vi "02-调小程序.vi"() -> ()   [LabVIEW 2015]
panel:
  out "数组":i32[](array[numeric])
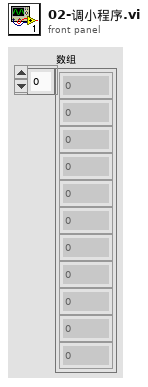
[diagram p1: front panel]
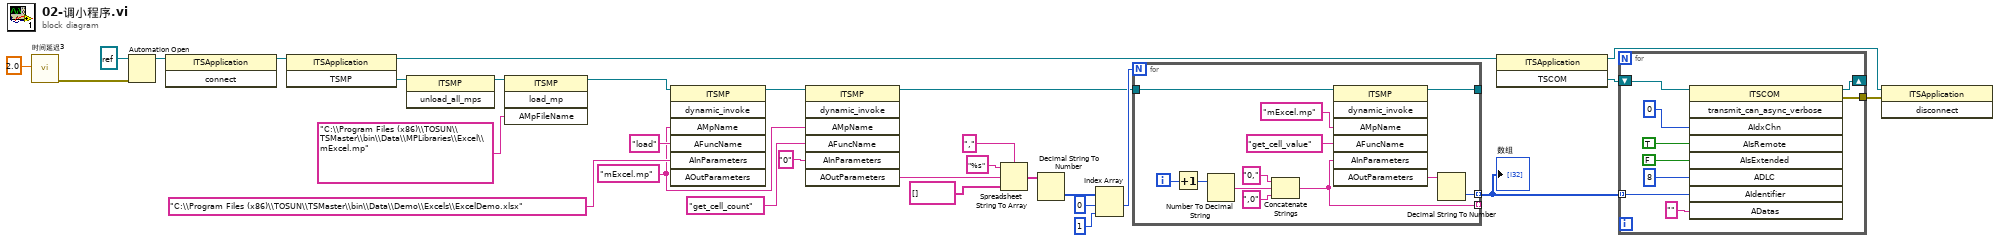
[diagram p0: block diagram]
diagram:
  w3 = "mExcel.mp" ("AMpName")
  n1 = call "时间延迟3"("Delay Time (s)"=2.0) -> ("error out"=w28:errorcluster)  [unwired: 10 in]
  n2 = Automation Open(error in (no error)=w28, Automation Refnum=refnum<k7> refnum ("TSMaster.ITSApplication")) -> (Automation Refnum=w27:refnum<k7>)  [unwired: 2 in, 1 out]
  n3 = invoke on="调用节点" class="ITSApplication" method="connect"(reference=w27) -> (reference out=w4:refnum<k7>)  [unwired: 2 in, 2 out]
  n4 = invoke on="调用节点" class="ITSApplication" method="TSMP"(reference=w4) -> (reference out=w6:refnum<k7>, "TSMP"=w23:refnum<k7>)  [unwired: 2 in, 1 out]
  n5 = invoke on="调用节点" class="ITSMP" method="unload_all_mps"(reference=w23) -> (reference out=w22:refnum<k7>)  [unwired: 2 in, 2 out]
  n6 = invoke on="调用节点" class="ITSMP" method="load_mp"(reference=w22, "AMpFileName"="C:\\Program Files (x86)\\TOSUN\\TSMaster\\bin\\Data\\MPLibraries\\Excel\\mExcel.mp") -> (reference out=w1:refnum<k7>)  [unwired: 2 in, 3 out]
  n7 = invoke on="调用节点" class="ITSMP" method="dynamic_invoke"(reference=w1, "AMpName"=w3, "AFuncName"="load", "AInParameters"="C:\\Program Files (x86)\\TOSUN\\TSMaster\\bin\\Data\\Demo\\Excels\\ExcelDemo.xlsx") -> (reference out=w2:refnum<k7>)  [unwired: 3 in, 6 out]
  n8 = invoke on="调用节点" class="ITSMP" method="dynamic_invoke"(reference=w2, "AMpName"=w3, "AFuncName"="get_cell_count", "AInParameters"="0") -> (reference out=w8:refnum<k7>, "AOutParameters"=w17:string)  [unwired: 3 in, 5 out]
  n9 = Spreadsheet String To Array(delimiter (Tab)="," ("分隔符(Tab)"), format string="%s" ("格式字符串"), spreadsheet string=w17, array type (2D Dbl)=string[] []) -> (array=w13:string[])
  n10 = Decimal String To Number(string=w13) -> (number=w12:i32[])  [unwired: 2 in, 1 out]
  n11 = Index Array(array=w12, index #1=0 ("索引"), index #2=1 ("索引")) -> (element #1=w9:i32)  [unwired: 1 out]
  n12 = for {
    N: w9 -> [_]
    tunnel: w8 -> [w40]
    tunnel: [w33] -> w26 mode=indexing
    tunnel: [w32] -> _
    tunnel: [w31] -> _ mode=indexing
    i -> [w38]
    n13 = Increment(x=w38) -> (x+1=w37:i32)
    n14 = Number To Decimal String(number=w37) -> (decimal integer string=w36:string)  [unwired: 1 in]
    n15 = Concatenate Strings("0," ("字符串"), w36, ",0" ("字符串")) -> (w31:string)
    n16 = invoke on="调用节点" class="ITSMP" method="dynamic_invoke"(reference=w40, "AMpName"="mExcel.mp", "AFuncName"="get_cell_value", "AInParameters"=w31) -> (reference out=w32:refnum<k7>, "AOutParameters"=w34:string)  [unwired: 3 in, 5 out]
    n17 = Decimal String To Number(string=w34) -> (number=w33:i32)  [unwired: 2 in, 1 out]
  }
  "数组" <- w26
  n18 = invoke on="调用节点" class="ITSApplication" method="TSCOM"(reference=w6) -> (reference out=w5:refnum<k7>, "TSCOM"=w25:refnum<k7>)  [unwired: 2 in, 1 out]
  n19 = for {
    shift-right: [w45] -> _
    shift-left: w25 -> [w51]
    tunnel: w26 -> [w44] mode=indexing
    tunnel: [w43] -> w24
    n20 = invoke on="调用节点" class="ITSCOM" method="transmit_can_async_verbose"(reference=w51, "AIdxChn"=0, "AIsRemote"=TRUE, "AIsExtended"=FALSE, "ADLC"=8, "AIdentifier"=w44, "ADatas"="") -> (reference out=w45:refnum<k7>, error out=w43:errorcluster)  [unwired: 2 in, 7 out]
  }
  n21 = invoke on="调用节点" class="ITSApplication" method="disconnect"(reference=w5, error in=w24) -> ()  [unwired: 1 in, 3 out]
